vi "mks946_sub_set.vi"(6 "error in (no error)":errorcluster, 7 "VISA_ref_in":refnum<visa-resource-name>="COM3", 9 "parameter":string="PR", 10 "command":string="PR", 11 "address":i32) -> (0 "status":bool, 2 "message":string, 3 "response":string, 4 "error out":errorcluster={"status"=TRUE, "code"=1, "source"="Scan From String (arg 1) in mks946_sub_get.vi"}, 5 "VISA_ref_out":refnum<visa-resource-name>="COM3")   [LabVIEW 2019]
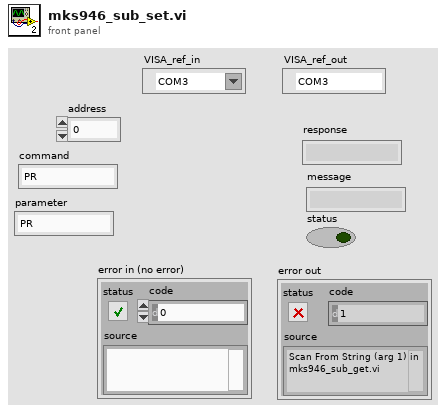
[diagram p1: front panel]
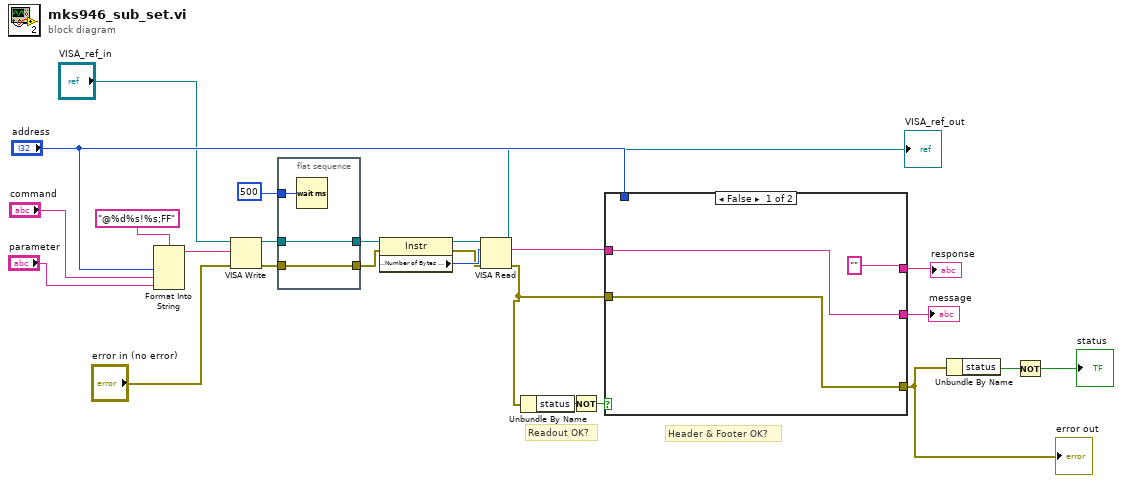
[diagram p0: block diagram]
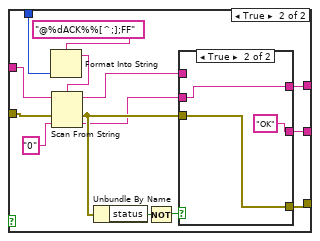
[diagram p2: hidden frame]
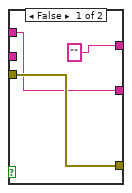
[diagram p3: hidden frame]
diagram:
  # "Header & Footer OK?"
  # "Readout OK?"
  n1 = Format Into String(format string="@%d%s!%s;FF", "address", "command", "parameter") -> (resulting string=w9:string)  [unwired: 2 in, 1 out]
  n2 = VISA Write(VISA resource name="VISA_ref_in", write buffer=w9, error in (no error)="error in (no error)") -> (VISA resource name out=w5:refnum<visa-resource-name>, error out=w4:errorcluster)  [unwired: 1 out]
  n3 = flat-sequence {
    tunnel: w4 -> [w27]
    tunnel: [w27] -> w14
    tunnel: w5 -> [w26]
    tunnel: [w26] -> w13
    tunnel: u32 500 ("mks946_delay") -> [w28]
    frame #0 {
      n4 = Wait (ms)(milliseconds to wait=w28) -> ()  [unwired: 1 out]
    }
  }
  n5 = property class="Instr"(reference=w13, error in=w14) -> (reference out=w22:refnum<visa-resource-name>, error out=w23:errorcluster, "Serial Settings:Number of Bytes at Serial Port"=w24:u32)
  n6 = VISA Read(VISA resource name=w22, byte count=w24, error in (no error)=w23) -> (VISA resource name out=→"VISA_ref_out":refnum<visa-resource-name>, read buffer=w16:string, error out=w17:errorcluster)  [unwired: 1 out]
  n7 = Unbundle By Name(w17) -> ("status"=w12:bool)
  n8 = Not(x=w12) -> (.not. x?=w15:bool)
  n9 = case shown="False" w15 {
    tunnel: [w31 w36] -> w20
    tunnel: w16 -> [w30 w45]
    tunnel: w17 -> [w31 w44]
    tunnel: "address" -> [_ w43]
    tunnel: ["" w33] -> w1
    tunnel: [w30 w32] -> w2
    frame False {
    }
    frame True {
      n10 = Format Into String(format string="@%dACK%%[^;];FF", w43) -> (resulting string=w42:string)  [unwired: 2 in, 1 out]
      n11 = Scan From String(format string=w42, input string=w45, error in=w44, default 1="0") -> (remaining string=w35:string, error out=w38:errorcluster, output 1=w37:string)  [unwired: 1 in, 1 out]
      n12 = Unbundle By Name(w38) -> ("status"=w40:bool)
      n13 = Not(x=w40) -> (.not. x?=w39:bool)
      n14 = case shown="True" w39 {
        tunnel: w38 -> [w48 w50]
        tunnel: w37 -> [_ w51]
        tunnel: [w48 w50] -> w36
        tunnel: w35 -> [w47 _]
        tunnel: ["" w51] -> w33
        tunnel: [w47 "OK"] -> w32
        frame False {
        }
        frame True {
        }
      }
    }
  }
  "error out" <- w20
  "response" <- w1
  "message" <- w2
  n15 = Unbundle By Name(w20) -> ("status"=w18:bool)
  n16 = Not(x=w18) -> (.not. x?=→"status":bool)
